vi "Convert Package Name (VIPM to NIPM).vi"(8 "error in (no error)":errorcluster, 9 "LabVIEW version in":string, 11 "VIPM Package Name":string) -> (0 "error out":errorcluster, 1 "LabVIEW version out":string, 3 "NIPM Package Name":string)   [LabVIEW 2014, in "vipm-to-nipm-package-converter.lvlib"]
doc: "Converts the VIPM package's Name to a LabVIEW-version specific NIPM Package Name. For example, \"oglib_string\" and \"18.0\" converts to \"oglib-string-lv-2014-32-bit\".\n\nINPUT(S):\n<b>LabVIEW version</b>: Specifies the LabVIEW version for the NIPM package to support (\"14.0\", \"14.0 (64-bit)\", \"18.0\", \"18.0 (64-bit)\", etc)"
uses:
  vipm-to-nipm-package-converter.lvlib
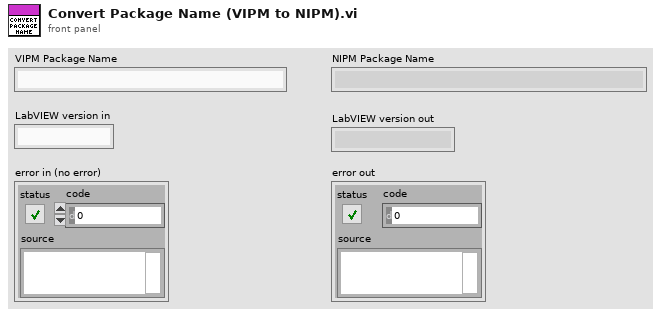
[diagram p1: front panel]
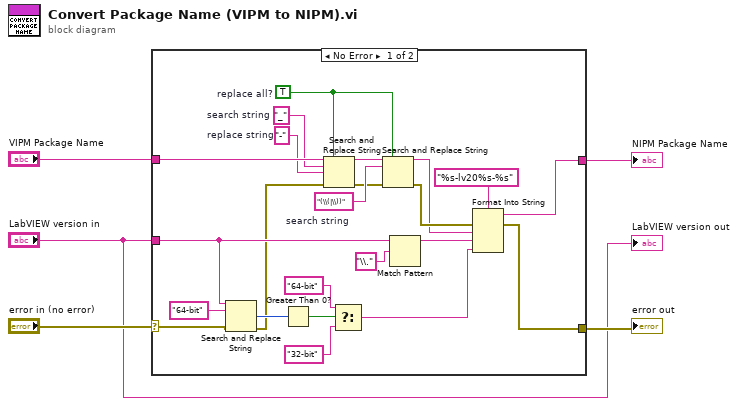
[diagram p0: block diagram]
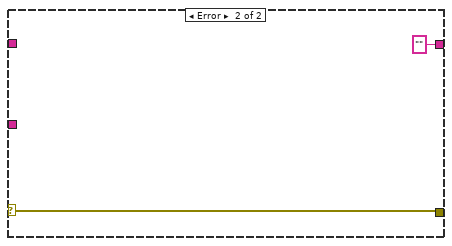
[diagram p2: hidden frame]
diagram:
  n1 = case shown="No Error" "error in (no error)" {
    selector: "error in (no error)" -> [w7 w29]
    tunnel: "VIPM Package Name" -> [w22 _]
    tunnel: [w19 w29] -> w3
    tunnel: [w18 ""] -> w2
    tunnel: "LabVIEW version in" -> [w9 _]
    frame No Error {
      w26 = "(\\(|\\))"  # search string
      w27 = TRUE  # replace all?
      w21 = "-"  # replace string
      w20 = "_"  # search string
      n2 = Search and Replace String(input string=w9, search string="64-bit", error in=w7) -> (number of replacements=w15:i32, error out=w6:errorcluster)  [unwired: 5 in, 2 out]
      n3 = Greater Than 0?(x=w15) -> (x > 0?=w14:bool)
      n4 = Search and Replace String(replace all?=w27, input string=w22, search string=w20, replace string=w21, error in=w6) -> (result string=w23:string, error out=w25:errorcluster)  [unwired: 3 in, 2 out]
      n5 = Select(t="64-bit" ("search string"), s=w14, f="32-bit" ("search string")) -> (s? t:f=w11:string)
      n6 = Search and Replace String(replace all?=w27, input string=w23, search string=w26, error in=w25) -> (result string=w24:string, error out=w28:errorcluster)  [unwired: 4 in, 2 out]
      n7 = Match Pattern(string=w9, regular expression="\\.") -> (before substring=w8:string)  [unwired: 1 in, 3 out]
      n8 = Format Into String(format string="%s-lv20%s-%s", error in=w28, w24, w8, w11) -> (resulting string=w18:string, error out=w19:errorcluster)  [unwired: 1 in]
    }
    frame Error {
    }
  }
  "error out" <- w3
  "NIPM Package Name" <- w2
  "LabVIEW version out" <- "LabVIEW version in"
